vi "pmu_Check Channel Error.vi"(8 "error in (no error)":errorcluster, 10 "physical channels":T2[](array[typedef]), 11 "phasor channels":T1[](array[typedef]) {"phasor unit scaling" max=16777215 format="%06x"; "phasor unit" items=["Voltage [V]"=0, "Current [A]"=16777216]}) -> (0 "error out":errorcluster)   [LabVIEW 2013, in "NI_EP_PMU.lvlib"]
uses:
  <vilib>/addons/Electrical Power/PMU/NI_EP_PMU.lvlib
  <vilib>/addons/Electrical Power/PMU/Common/Controls/pmu_Physical Channel.ctl
  <vilib>/addons/Electrical Power/PMU/Common/Controls/pmu_Channel Phase.ctl
  <vilib>/addons/Electrical Power/PMU/Common/Controls/pmu_Phasor Channel.ctl
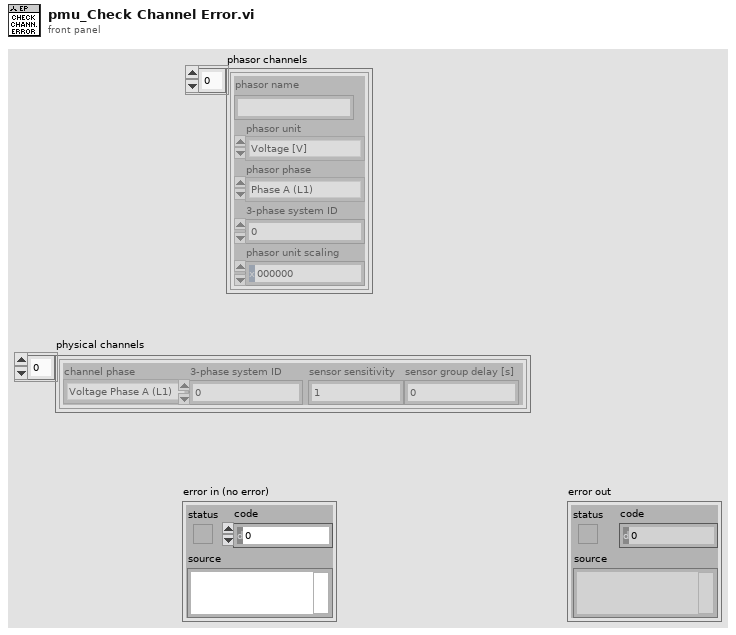
[diagram p1: front panel]
types:
  T1 = typedef "NI_EP_PMU.lvlib/pmu_Phasor Channel.ctl" = cluster{"phasor name":string, "phasor unit":u32, "phasor phase":enum16{"Phase A (L1)", "Phase B (L2)", "Phase C (L3)", "Phase N", "Positive sequence", "Negative sequence", "Zero sequence"}, "3-phase system ID":u8, "phasor unit scaling":u32}
  T2 = typedef "NI_EP_PMU.lvlib/pmu_Physical Channel.ctl" = cluster{"channel phase":T3, "3-phase system ID":u8, "sensor sensitivity":dbl, "sensor group delay [s]":dbl}
  T3 = typedef "NI_EP_PMU.lvlib/pmu_Channel Phase.ctl" = enum16{"Voltage Phase A (L1)", "Voltage Phase B (L2)", "Voltage Phase C (L3)", "Voltage Phase N (Neutral)", "Current Phase A (L1)", "Current Phase B (L2)", "Current Phase C (L3)", "Current Phase N (Neutral)"}
  T4 = cluster{"3-phase system ID":u8, "channel phase":T3}[]
  T5 = enum16{"Phase A (L1)", "Phase B (L2)", "Phase C (L3)", "Phase N", "Positive sequence", "Negative sequence", "Zero sequence"}
  T6 = cluster{"3-phase system ID":u8, "channel phase":T3}
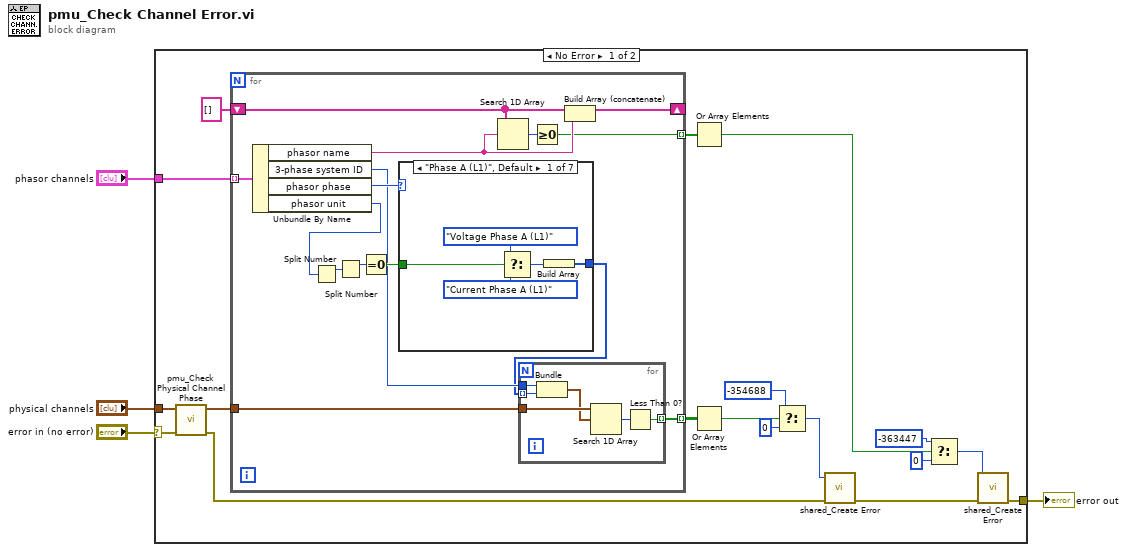
[diagram p0: block diagram]
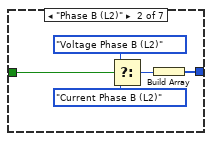
[diagram p2: hidden frame]
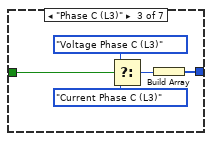
[diagram p3: hidden frame]
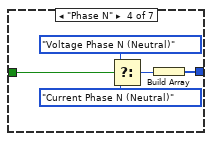
[diagram p4: hidden frame]
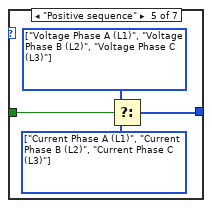
[diagram p5: hidden frame]
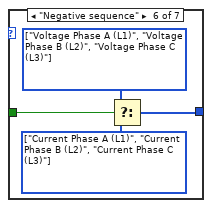
[diagram p6: hidden frame]
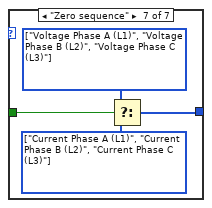
[diagram p7: hidden frame]
diagram:
  n1 = case shown="No Error" "error in (no error)" {
    selector: "error in (no error)" -> [w7 w76]
    tunnel: "physical channels" -> [w8 _]
    tunnel: [w9 w76] -> w2
    tunnel: "phasor channels" -> [w17 _]
    frame No Error {
      n2 = call <vilib>:"pmu_Check Physical Channel Phase.vi"("error in (no error)"=w7, "physical channels in"=w8) -> ("error out"=w6:errorcluster, "Array"=w5:T4)  [unwired: 8 in]
      n3 = for {
        tunnel: w17 -> [w37] mode=indexing
        shift-right: [w34] -> _
        shift-left: string[] [] -> [w33]
        tunnel: [w32] -> w22 mode=indexing
        tunnel: w5 -> [w27]
        tunnel: [w23] -> w19 mode=indexing
        n4 = Unbundle By Name(w37) -> ("phasor name"=w35:string, "3-phase system ID"=w25:u8, "phasor phase"=w31:T5, "phasor unit"=w26:u32)
        n5 = Split Number(x=w26) -> (hi(x)=w30:u16)  [unwired: 1 out]
        n6 = Split Number(x=w30) -> (hi(x)=w29:u8)  [unwired: 1 out]
        n7 = Equal To 0?(x=w29) -> (x = 0?=w28:bool)
        n8 = case shown="\"Phase A (L1)\", Default" w31 {
          tunnel: w28 -> [w46 w51 w56 w61 w67 w71 w75]
          tunnel: [w44 w49 w54 w59 w66 w70 w74] -> w24
          frame "Phase A (L1)", Default {
            n9 = Select(t=pmu_Channel_Phase."Voltage Phase A (L1)" ("channel phase"), s=w46, f=pmu_Channel_Phase."Current Phase A (L1)" ("channel phase")) -> (s? t:f=w45:T3)
            n10 = Build Array(w45) -> (w44:T3[])
          }
          frame "Phase B (L2)" {
            n11 = Select(t=pmu_Channel_Phase."Voltage Phase B (L2)" ("channel phase"), s=w51, f=pmu_Channel_Phase."Current Phase B (L2)" ("channel phase")) -> (s? t:f=w50:T3)
            n12 = Build Array(w50) -> (w49:T3[])
          }
          frame "Phase C (L3)" {
            n13 = Select(t=pmu_Channel_Phase."Voltage Phase C (L3)" ("channel phase"), s=w56, f=pmu_Channel_Phase."Current Phase C (L3)" ("channel phase")) -> (s? t:f=w55:T3)
            n14 = Build Array(w55) -> (w54:T3[])
          }
          frame "Phase N" {
            n15 = Select(t=pmu_Channel_Phase."Voltage Phase N (Neutral)" ("channel phase"), s=w61, f=pmu_Channel_Phase."Current Phase N (Neutral)" ("channel phase")) -> (s? t:f=w60:T3)
            n16 = Build Array(w60) -> (w59:T3[])
          }
          frame "Positive sequence" {
            w65 = T3[] [enum."Current Phase A (L1)", enum."Current Phase B (L2)", enum."Current Phase C (L3)"] items=["Voltage Phase A (L1)", "Voltage Phase B (L2)", "Voltage Phase C (L3)", "Voltage Phase N (Neutral)", "Current Phase A (L1)", "Current Phase B (L2)", "Current Phase C (L3)", "Current Phase N (Neutral)"]
            w64 = T3[] [enum."Voltage Phase A (L1)", enum."Voltage Phase B (L2)", enum."Voltage Phase C (L3)"] items=["Voltage Phase A (L1)", "Voltage Phase B (L2)", "Voltage Phase C (L3)", "Voltage Phase N (Neutral)", "Current Phase A (L1)", "Current Phase B (L2)", "Current Phase C (L3)", "Current Phase N (Neutral)"]
            n17 = Select(t=w64, s=w67, f=w65) -> (s? t:f=w66:T3[])
          }
          frame "Negative sequence" {
            w69 = T3[] [enum."Current Phase A (L1)", enum."Current Phase B (L2)", enum."Current Phase C (L3)"] items=["Voltage Phase A (L1)", "Voltage Phase B (L2)", "Voltage Phase C (L3)", "Voltage Phase N (Neutral)", "Current Phase A (L1)", "Current Phase B (L2)", "Current Phase C (L3)", "Current Phase N (Neutral)"]
            w68 = T3[] [enum."Voltage Phase A (L1)", enum."Voltage Phase B (L2)", enum."Voltage Phase C (L3)"] items=["Voltage Phase A (L1)", "Voltage Phase B (L2)", "Voltage Phase C (L3)", "Voltage Phase N (Neutral)", "Current Phase A (L1)", "Current Phase B (L2)", "Current Phase C (L3)", "Current Phase N (Neutral)"]
            n18 = Select(t=w68, s=w71, f=w69) -> (s? t:f=w70:T3[])
          }
          frame "Zero sequence" {
            w73 = T3[] [enum."Current Phase A (L1)", enum."Current Phase B (L2)", enum."Current Phase C (L3)"] items=["Voltage Phase A (L1)", "Voltage Phase B (L2)", "Voltage Phase C (L3)", "Voltage Phase N (Neutral)", "Current Phase A (L1)", "Current Phase B (L2)", "Current Phase C (L3)", "Current Phase N (Neutral)"]
            w72 = T3[] [enum."Voltage Phase A (L1)", enum."Voltage Phase B (L2)", enum."Voltage Phase C (L3)"] items=["Voltage Phase A (L1)", "Voltage Phase B (L2)", "Voltage Phase C (L3)", "Voltage Phase N (Neutral)", "Current Phase A (L1)", "Current Phase B (L2)", "Current Phase C (L3)", "Current Phase N (Neutral)"]
            n19 = Select(t=w72, s=w75, f=w73) -> (s? t:f=w74:T3[])
          }
        }
        n20 = Search 1D Array(1D array=w33, element=w35) -> (index of element=w36:i32)  [unwired: 1 in]
        n21 = for {
          tunnel: w27 -> [w43]
          tunnel: w25 -> [w42]
          tunnel: w24 -> [w41] mode=indexing
          tunnel: [w38] -> w23 mode=indexing
          n22 = Bundle("3-phase system ID"=w42, "channel phase"=w41) -> (w40:T6)  [unwired: 1 in]
          n23 = Search 1D Array(1D array=w43, element=w40) -> (index of element=w39:i32)  [unwired: 1 in]
          n24 = Less Than 0?(x=w39) -> (x < 0?=w38:bool)
        }
        n25 = Greater Or Equal To 0?(x=w36) -> (x >= 0?=w32:bool)
        n26 = Build Array (concatenate)(w33, w35) -> (w34:string[])
      }
      n27 = Or Array Elements(Boolean array=w22) -> (logical OR=w20:bool)
      n28 = Or Array Elements(Boolean array=w19) -> (logical OR=w18:bool)
      n29 = Select(t=-354688 ("error code (0)"), s=w18, f=0 ("error code (0)")) -> (s? t:f=w14:i32)
      n30 = call <vilib>:"shared_Create Error.vi"("error in (no error)"=w6, "error code (0)"=w14) -> ("error out"=w10:errorcluster)  [unwired: 9 in]
      n31 = Select(t=-363447 ("error code (0)"), s=w20, f=0 ("error code (0)")) -> (s? t:f=w11:i32)
      n32 = call <vilib>:"shared_Create Error.vi"("error in (no error)"=w10, "error code (0)"=w11) -> ("error out"=w9:errorcluster)  [unwired: 9 in]
    }
    frame Error {
    }
  }
  "error out" <- w2
